vi "Newport_PM_Autorange_Enable.vi"(7 "DUT Count":i32=1 min=1 max=8 step=1, 8 "Error In":errorcluster, 11 "Reference In":refnum<k24>) -> (0 "Error Out":errorcluster, 1 "Query Response":string, 2 "Auto Range Enabled":bool, 3 "Reference Out":refnum<k24>)   [LabVIEW 2017]
uses:
  C:/Program Files (x86)/Newport/Newport USB Driver/Bin/UsbDllWrap.dll
  Program Files (x86)/Newport/Newport USB Driver/Bin/UsbDllWrap.dll
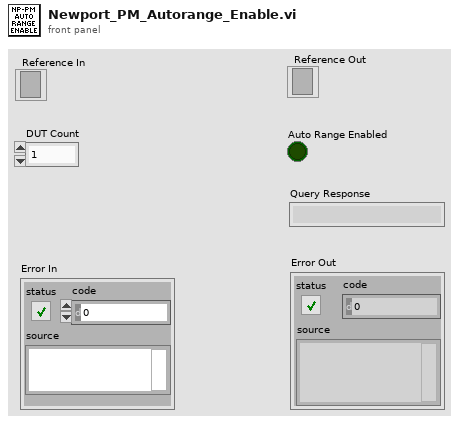
[diagram p1: front panel]
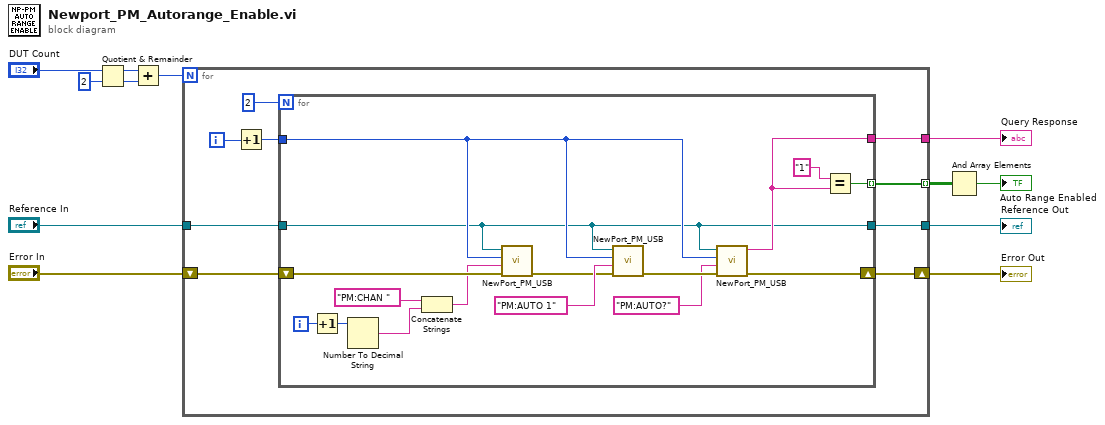
[diagram p0: block diagram]
diagram:
  n1 = Quotient & Remainder(x="DUT Count", y=2) -> (x-y*floor(x/y)=w6:i32, floor(x/y)=w7:i32)
  n2 = Add(x=w6, y=w7) -> (x+y=w5:i32)
  n3 = for {
    N: w5 -> [_]
    tunnel: "Reference In" -> [w17]
    shift-right: [w21] -> w11
    shift-left: "Error In" -> [w15]
    tunnel: [w19] -> w4 mode=indexing
    tunnel: [w18] -> w2
    tunnel: [w13] -> w1
    i -> [w20]
    n4 = Increment(x=w20) -> (x+1=w16:i32)
    n5 = for {
      N: 2 -> [_]
      tunnel: [w33] -> w19 mode=indexing
      tunnel: [w32] -> w18
      tunnel: w17 -> [w22]
      tunnel: w16 -> [w30]
      shift-right: [w36] -> w21
      shift-left: w15 -> [w29]
      tunnel: [w22] -> w13
      i -> [w23]
      n6 = Increment(x=w23) -> (x+1=w24:i32)
      n7 = Number To Decimal String(number=w24) -> (decimal integer string=w25:string)  [unwired: 1 in]
      n8 = Concatenate Strings("PM:CHAN " ("PM:CMD_QUERY In"), w25) -> (w26:string)
      n9 = call "NewPort_PM_USB.vi"("error in"=w29, "PM:CMD_QUERY In"=w26, "USB Address"=w30, "reference"=w22) -> ("error out"=w28:errorcluster)  [unwired: 5 in, 2 out]
      n10 = call "NewPort_PM_USB.vi"("error in"=w28, "PM:CMD_QUERY In"="PM:AUTO 1", "USB Address"=w30, "reference"=w22) -> ("error out"=w37:errorcluster)  [unwired: 5 in, 2 out]
      n11 = call "NewPort_PM_USB.vi"("error in"=w37, "PM:CMD_QUERY In"="PM:AUTO?", "USB Address"=w30, "reference"=w22) -> ("error out"=w36:errorcluster, "Query-String\nfrom Read Buffer\nComplete Info"=w32:string)  [unwired: 5 in, 1 out]
      n12 = Equal?(x="1" ("y"), y=w32) -> (x = y?=w33:bool)
    }
  }
  "Error Out" <- w11
  "Query Response" <- w2
  "Reference Out" <- w1
  n13 = And Array Elements(Boolean array=w4) -> (logical AND=→"Auto Range Enabled":bool)
